vi "力特性 对称性.vi"(8 "油压B":dbl[](array[numeric]), 9 "油压A":dbl[](array[numeric]), 10 "扭矩B":dbl[](array[numeric]), 11 "扭矩A":dbl[](array[numeric])) -> (3 "对称性":dbl)   [LabVIEW 2015, in "Logging.lvlib"]
uses:
  Logging.lvlib
  <vilib>/Analysis/1siggen.llb/Ramp Pattern by Samples.vi
  <vilib>/gmath/NI_Gmath.lvlib
  <vilib>/Analysis/NI_AALBase.lvlib
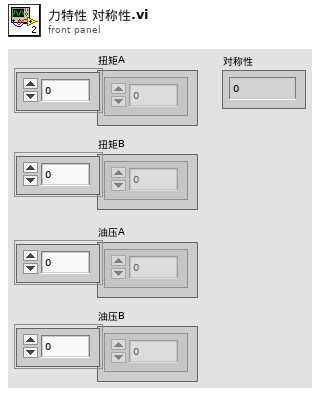
[diagram p1: front panel]
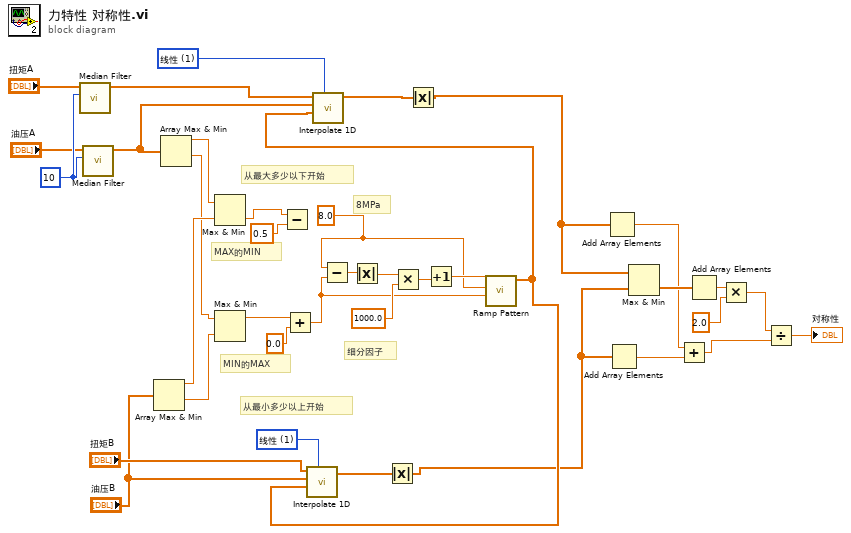
[diagram p0: block diagram]
diagram:
  w7 = 10 ("left rank")
  w11 = 8.0 ("x")
  w24 = 1 items=["最近", "线性", "样条", "cubic Hermite", "拉格朗日"] ("method")
  w37 = 1 items=["最近", "线性", "样条", "cubic Hermite", "拉格朗日"] ("method")
  # "8MPa"
  # "细分因子"
  # "从最大多少以下开始"
  # "从最小多少以上开始"
  # "MIN的MAX"
  # "MAX的MIN"
  n1 = call <vilib>:"Median Filter.vi"("left rank"=w7, "X"="扭矩A") -> ("Filtered X"=w2:dbl[])  [unwired: 8 in, 1 out]
  n2 = call <vilib>:"Median Filter.vi"("left rank"=w7, "X"="油压A") -> ("Filtered X"=w1:dbl[])  [unwired: 8 in, 1 out]
  n3 = Array Max & Min(array="油压B") -> (max value=w35:dbl, min value=w33:dbl)  [unwired: 2 out]
  n4 = Array Max & Min(array=w1) -> (max value=w36:dbl, min value=w34:dbl)  [unwired: 2 out]
  n5 = Max & Min(x=w36, y=w35) -> (min(x,y)=w20:dbl)  [unwired: 1 out]
  n6 = Max & Min(x=w34, y=w33) -> (max(x,y)=w21:dbl)  [unwired: 1 out]
  n7 = Subtract(x=w20, y=0.5) -> ()  [unwired: 1 out]
  n8 = Add(x=w21, y=0.0) -> (x+y=w25:dbl)
  n9 = Subtract(x=w11, y=w25) -> (x-y=w30:dbl)
  n10 = Absolute Value(x=w30) -> (abs(x)=w28:dbl)
  n11 = Multiply(x=w28, y=1000.0) -> (x*y=w29:dbl)
  n12 = Increment(x=w29) -> (x+1=w26:dbl)
  n13 = call-poly <vilib>:"Ramp Pattern.vi"("start"=w25, "end"=w11, "samples"=w26) -> ("Ramp Pattern"=w9:dbl[])  [unwired: 7 in, 1 out]
  n14 = call <vilib>:"Interpolate 1D.vi"("method"=w24, "xi"=w9, "X"="油压B", "Y"="扭矩B") -> ("yi"=w4:dbl[])  [unwired: 5 in, 2 out]
  n15 = call <vilib>:"Interpolate 1D.vi"("method"=w37, "xi"=w9, "X"=w1, "Y"=w2) -> ("yi"=w8:dbl[])  [unwired: 5 in, 2 out]
  n16 = Absolute Value(x=w4) -> (abs(x)=w3:dbl[])
  n17 = Absolute Value(x=w8) -> (abs(x)=w10:dbl[])
  n18 = Add Array Elements(numeric array=w10) -> (sum=w17:dbl)
  n19 = Add Array Elements(numeric array=w3) -> (sum=w18:dbl)
  n20 = Max & Min(x=w10, y=w3) -> (min(x,y)=w19:dbl[])  [unwired: 1 out]
  n21 = Add(x=w17, y=w18) -> (x+y=w13:dbl)
  n22 = Add Array Elements(numeric array=w19) -> (sum=w16:dbl)
  n23 = Multiply(x=w16, y=2.0) -> (x*y=w14:dbl)
  n24 = Divide(x=w14, y=w13) -> (x/y=→"对称性":dbl)
